vi "Read from Coils DB.vi"(8 "error in (no error)":errorcluster, 9 "Length (-1)":i32=-1, 10 "Modbus Address":u16, 11 "MB Data Block in":refnum<class "MB Data Block.lvclass">) -> (0 "error out":errorcluster, 2 "Data out":bool[](array[boolean]), 3 "MB Data Block out":refnum<class "MB Data Block.lvclass">)   [LabVIEW 2018, in "MB PLC Client.lvlib" / "MB Data Block.lvclass"]
uses:
  MB Data Block.lvclass
  MB Data Block.lvclass/MB Data Block.ctl
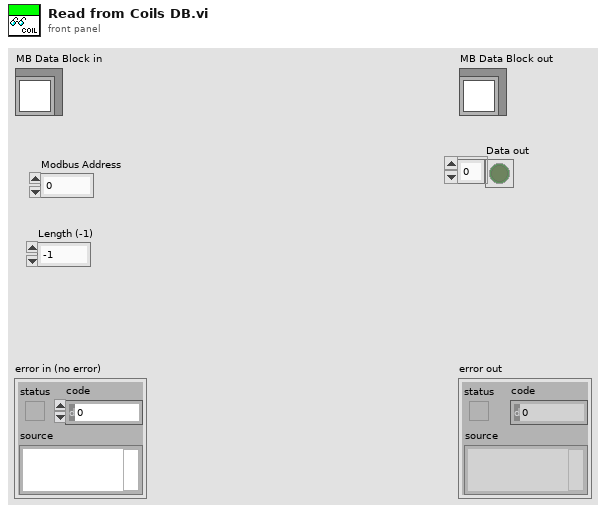
[diagram p1: front panel]
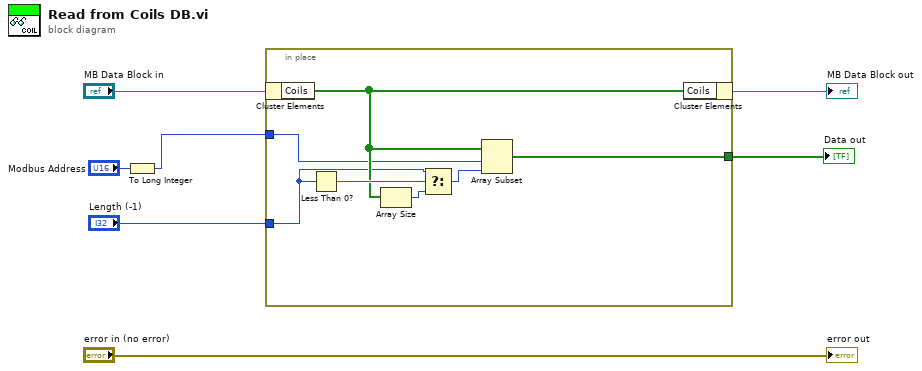
[diagram p0: block diagram]
diagram:
  n1 = To Long Integer(number="Modbus Address") -> (32bit integer=w3:i32)
  n2 = in-place {
    in-place-border: w3 -> [w10]
    in-place-border: "Length (-1)" -> [w9]
    in-place-border: [w8] -> w1
    n3 = in-place-cluster #1("MB Data Block in") -> ("Coils"=w11:bool[])
    n4 = Less Than 0?(x=w9) -> (x < 0?=w13:bool)
    n5 = Array Size(array=w11) -> (size(s)=w14:i32)
    n6 = Select(t=w9, s=w13, f=w14) -> (s? t:f=w12:i32)
    n7 = Array Subset(array=w11, index=w10, length=w12) -> (w8:bool[])
    n8 = in-place-cluster #1("Coils"=w11) -> (→"MB Data Block out":refnum<class "MB Data Block.lvclass">)
  }
  "Data out" <- w1
  "error out" <- "error in (no error)"
